vi "Roll Pitch Yaw to Rotation Matrix.vi"(1 "angles":cluster{"roll":dbl, "pitch":dbl, "yaw":dbl}) -> (0 "rotation matrix":T1)   [LabVIEW 2017, in "NI_Kinematics.lvlib"]
doc: "Converts <B>roll</B>, <B>pitch</B>, and <B>yaw</B> angles to the corresponding <B>rotation matrix</B>.\n\n<B>.m file:</B> rpy2r"
uses:
  <vilib>/robotics/Kinematics/NI_Kinematics.lvlib
  <vilib>/Analysis/Matrix/Datatypes/RealMatrix.ctl
  <vilib>/Analysis/baseanly.llb/Real A x B.vi
  <vilib>/Analysis/NI_AALBase.lvlib
  <vilib>/Analysis/Matrix/NI_Matrix.lvlib
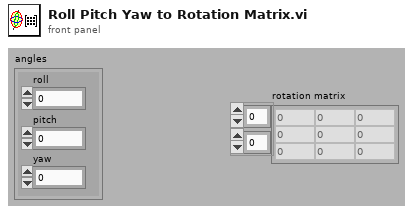
[diagram p1: front panel]
types:
  T1 = typedef "NI_Matrix.lvlib/RealMatrix.ctl" = dbl[][]
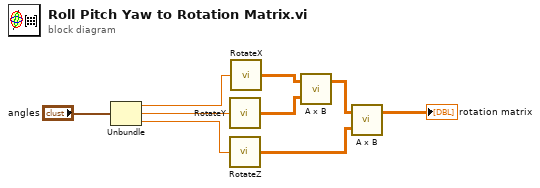
[diagram p0: block diagram]
diagram:
  n1 = Unbundle("angles") -> ("roll"=w8:dbl, "pitch"=w7:dbl, "yaw"=w6:dbl)
  n2 = call <vilib>:"RotateY.vi"("theta"=w7) -> ("rotation matrix"=w4:T1)
  n3 = call <vilib>:"RotateZ.vi"("theta"=w6) -> ("rotation matrix"=w3:T1)
  n4 = call <vilib>:"RotateX.vi"("theta"=w8) -> ("rotation matrix"=w5:T1)
  n5 = call-poly <vilib>:"A x B.vi"("B"=w4, "A"=w5) -> ("A x B"=w2:T1)  [unwired: 1 out]
  n6 = call-poly <vilib>:"A x B.vi"("B"=w3, "A"=w2) -> ("A x B"=→"rotation matrix":T1)  [unwired: 1 out]
